vi "revert direction.vi"(8 "error in (no error)":errorcluster, 11 "Autofocus in":refnum<class "Autofocus.lvclass">) -> (0 "error out":errorcluster, 3 "Autofocus out":refnum<class "Autofocus.lvclass">)   [LabVIEW 2012, in "Autofocus.lvclass"]
uses:
  Autofocus.lvclass
  Autofocus.lvclass/Autofocus.ctl
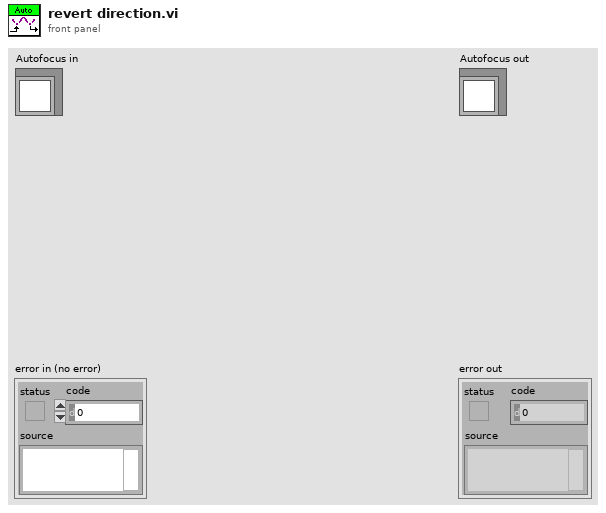
[diagram p1: front panel]
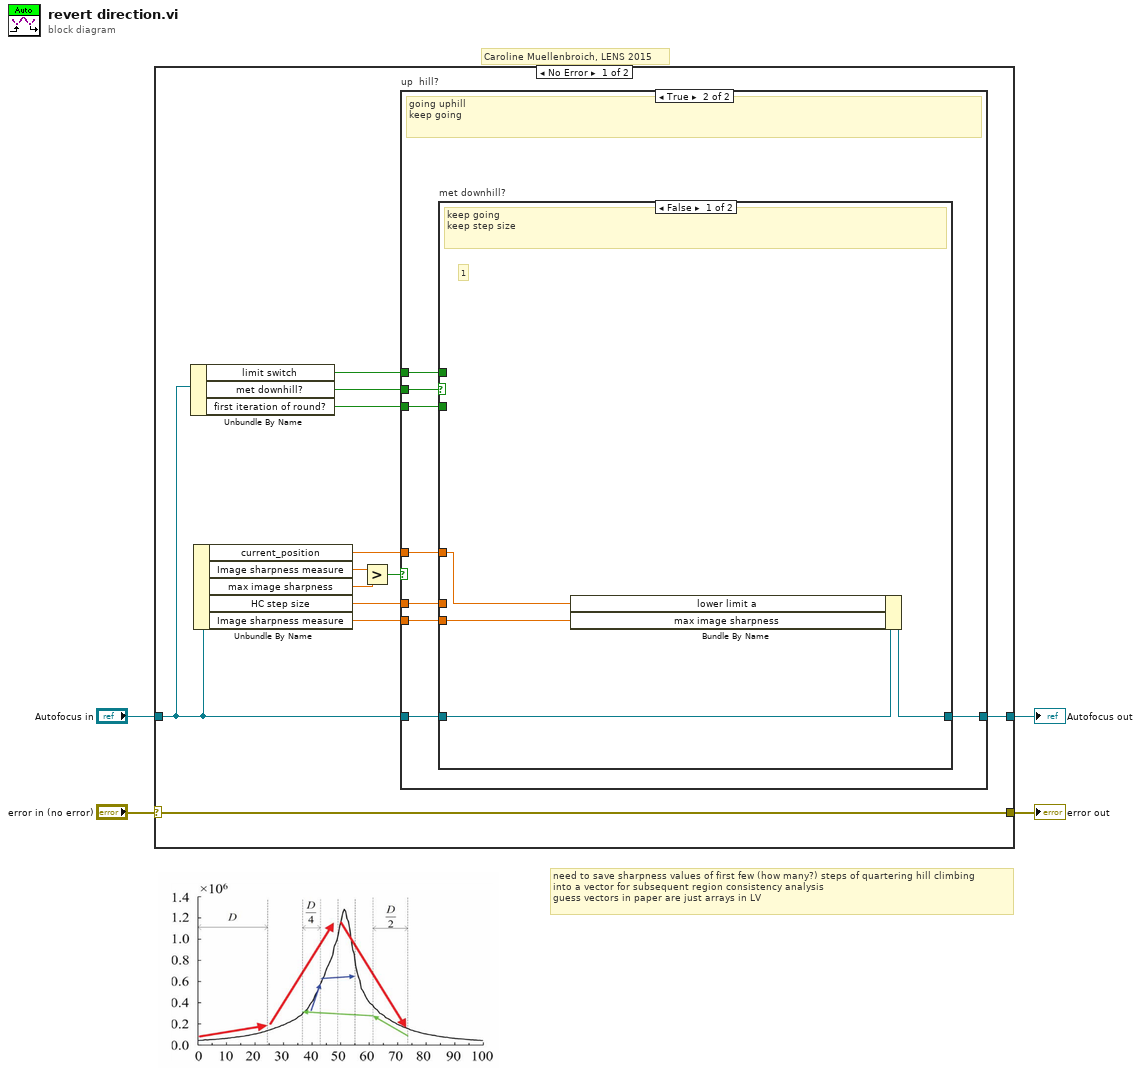
[diagram p0: block diagram]
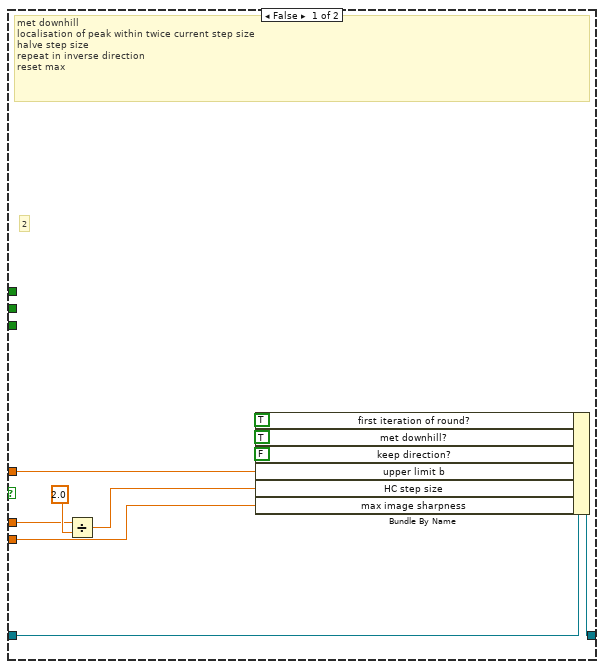
[diagram p2: hidden frame]
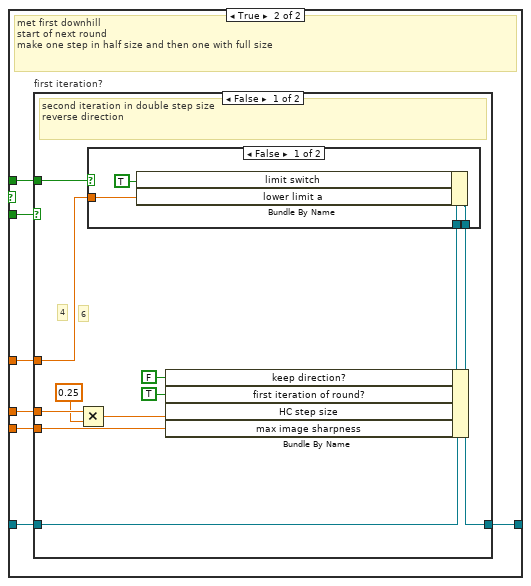
[diagram p3: hidden frame]
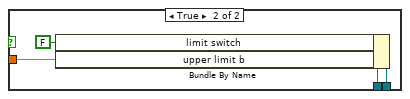
[diagram p4: hidden frame]
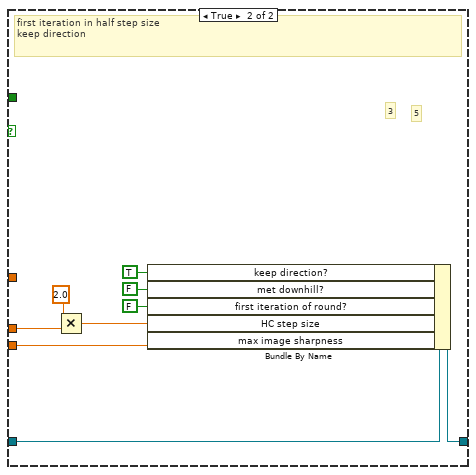
[diagram p5: hidden frame]
diagram:
  # "need to save sharpness values of first few (how many?) steps of quartering hill climbing\ninto a vector for subsequent region consistency analysis\nguess vectors in paper are just arrays in LV"
  # "Caroline Muellenbroich, LENS 2015"
  n1 = case shown="No Error" "error in (no error)" {
    selector: "error in (no error)" -> [w16 w75]
    tunnel: [w16 w75] -> w3
    tunnel: [w12 w74] -> w1
    tunnel: "Autofocus in" -> [w8 w74]
    frame No Error {
      n2 = Unbundle By Name(w8) -> ("limit switch"=w7:bool, "met downhill?"=w6:bool, "first iteration of round?"=w5:bool)
      n3 = Unbundle By Name(w8) -> ("current_position"=w9:dbl, "Image sharpness measure"=w15:dbl, "max image sharpness"=w14:dbl, "HC step size"=w11:dbl, "Image sharpness measure"=w10:dbl)
      n4 = Greater?(x=w15, y=w14) -> (0:w13:bool)
      n5 = case "up  hill?" shown="True" w13 {
        tunnel: w8 -> [w26 w33]
        tunnel: [w25 w32] -> w12
        tunnel: w11 -> [w23 w30]
        tunnel: w10 -> [w21 w31]
        tunnel: w6 -> [_ w34]
        tunnel: w5 -> [_ w29]
        tunnel: w9 -> [w20 w28]
        tunnel: w7 -> [_ w27]
        frame False {
          # "2"
          # "met downhill\nlocalisation of peak within twice current step size\nhalve step size\nrepeat in inverse direction\nreset max"
          n6 = Divide(x=w23, y=2.0) -> (x/y=w22:dbl)
          n7 = Bundle By Name(cluster=w26, "first iteration of round?"=TRUE ("Runtime cluster.Hill Climbing.first iteration of round?"), "met downhill?"=TRUE ("Runtime cluster.Hill Climbing.met downhill?"), "keep direction?"=FALSE ("Runtime cluster.Hill Climbing.keep direction?"), "upper limit b"=w20, "HC step size"=w22, "max image sharpness"=w21) -> (w25:refnum<class "Autofocus.lvclass">)
        }
        frame True {
          # "going uphill\nkeep going"
          n8 = case "met downhill?" shown="False" w34 {
            tunnel: w33 -> [w38 w43]
            tunnel: [w37 w42] -> w32
            tunnel: w31 -> [w36 w41]
            tunnel: w30 -> [_ w45]
            tunnel: w29 -> [_ w44]
            tunnel: w28 -> [w35 w40]
            tunnel: w27 -> [_ w39]
            frame False {
              # "1"
              # "keep going \nkeep step size"
              n9 = Bundle By Name(cluster=w38, "lower limit a"=w35, "max image sharpness"=w36) -> (w37:refnum<class "Autofocus.lvclass">)
            }
            frame True {
              # "met first downhill\nstart of next round\nmake one step in half size and then one with full size"
              n10 = case "first iteration?" shown="False" w44 {
                tunnel: w45 -> [w53 w69]
                tunnel: w43 -> [w56 w73]
                tunnel: [w48 w72] -> w42
                tunnel: w41 -> [w54 w71]
                tunnel: w40 -> [w49 _]
                tunnel: w39 -> [w50 _]
                frame False {
                  # "6"
                  # "4"
                  # "second iteration in double step size\nreverse direction"
                  n11 = Multiply(x=w53, y=0.25) -> (x*y=w55:dbl)
                  n12 = Bundle By Name(cluster=w56, "keep direction?"=FALSE ("Runtime cluster.Hill Climbing.keep direction?"), "first iteration of round?"=TRUE ("Runtime cluster.Hill Climbing.first iteration of round?"), "HC step size"=w55, "max image sharpness"=w54) -> (w51:refnum<class "Autofocus.lvclass">)
                  n13 = case shown="False" w50 {
                    tunnel: [w60 w64] -> w48
                    tunnel: w51 -> [w59 w63]
                    tunnel: w49 -> [w58 w62]
                    frame False {
                      n14 = Bundle By Name(cluster=w59, "limit switch"=TRUE ("Runtime cluster.limit switch"), "lower limit a"=w58) -> (w60:refnum<class "Autofocus.lvclass">)
                    }
                    frame True {
                      n15 = Bundle By Name(cluster=w63, "limit switch"=FALSE ("Runtime cluster.limit switch"), "upper limit b"=w62) -> (w64:refnum<class "Autofocus.lvclass">)
                    }
                  }
                }
                frame True {
                  # "5"
                  # "3"
                  # "first iteration in half step size\nkeep direction"
                  n16 = Multiply(x=2.0, y=w69) -> (x*y=w68:dbl)
                  n17 = Bundle By Name(cluster=w73, "keep direction?"=TRUE ("Runtime cluster.Hill Climbing.keep direction?"), "met downhill?"=FALSE ("Runtime cluster.Hill Climbing.met downhill?"), "first iteration of round?"=FALSE ("Runtime cluster.first iteration of round?"), "HC step size"=w68, "max image sharpness"=w71) -> (w72:refnum<class "Autofocus.lvclass">)
                }
              }
            }
          }
        }
      }
    }
    frame Error {
    }
  }
  "error out" <- w3
  "Autofocus out" <- w1
